vi "set_Xscale_range.vi"(8 "error in (no error)":errorcluster, 11 "Detector in":refnum<class "Detector.lvclass">) -> (0 "error out":errorcluster, 3 "Detector out":refnum<class "Detector.lvclass">)   [LabVIEW 2015, in "Detector.lvclass"]
uses:
  Detector.lvclass
  Detector.lvclass/Detector.ctl
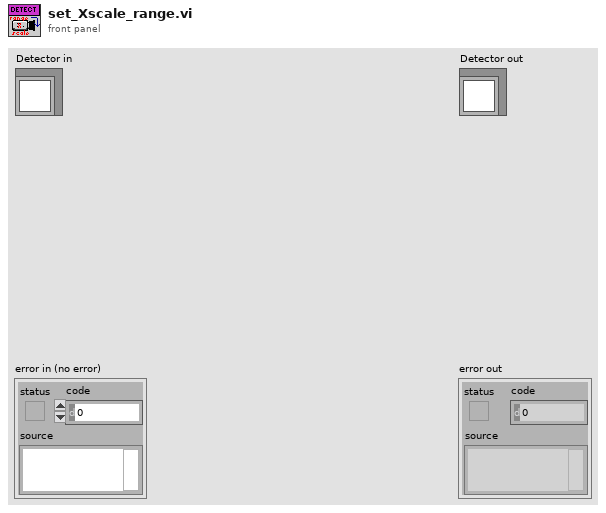
[diagram p1: front panel]
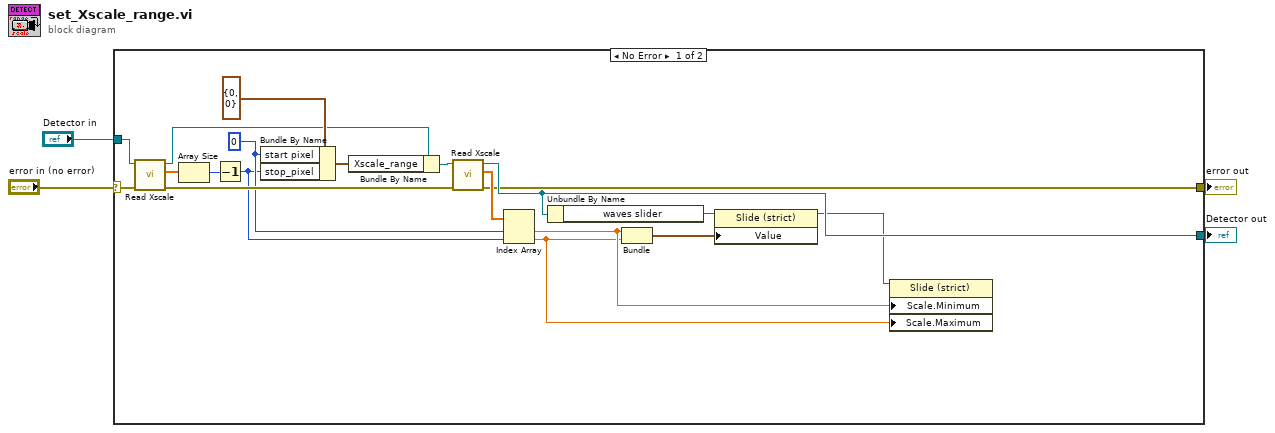
[diagram p0: block diagram]
diagram:
  n1 = case shown="No Error" "error in (no error)" {
    selector: "error in (no error)" -> [w22 w24]
    tunnel: [w8 w24] -> w3
    tunnel: [w9 w25] -> w1
    tunnel: "Detector in" -> [w23 w25]
    frame No Error {
      w12 = 0 ("start pixel")
      n2 = call "Read Xscale.vi"("error in (no error)"=w22, "Detector en entrée"=w23) -> ("error out"=w15:errorcluster, "Xscale"=w21:dbl[], "Detector en sortie"=w18:refnum<class "Detector.lvclass">)  [unwired: 7 in]
      n3 = Array Size(array=w21) -> (size(s)=w19:i32)
      n4 = Decrement(x=w19) -> (x-1=w11:i32)
      n5 = Bundle By Name(cluster=cluster{"start pixel":i32, "stop_pixel":i32} {"start pixel"=0, "stop_pixel"=0} ("Xscale_range"), "start pixel"=w12, "stop_pixel"=w11) -> (w16:cluster{"start pixel":i32, "stop_pixel":i32})
      n6 = Bundle By Name(cluster=w18, "Xscale_range"=w16) -> (w14:refnum<class "Detector.lvclass">)
      n7 = call "Read Xscale.vi"("error in (no error)"=w15, "Detector en entrée"=w14) -> ("error out"=w8:errorcluster, "Xscale"=w13:dbl[], "Detector en sortie"=w9:refnum<class "Detector.lvclass">)  [unwired: 7 in]
      n8 = Index Array(array=w13, index #1=w12, index #2=w11) -> (element #1=w6:dbl, element #2=w5:dbl)
      n9 = Unbundle By Name(w9) -> ("waves slider"=w17:refnum<vi>)
      n10 = Bundle("Numérique"=w6, "Numérique"=w5) -> (w10:cluster{"Numérique":dbl, "Numérique":dbl})  [unwired: 1 in]
      n11 = property class="Slide (strict)"(reference=w17, "Value"=w10) -> (reference out=w7:refnum<vi>)  [unwired: 1 in, 1 out]
      n12 = property class="Slide (strict)"(reference=w7, "Scale.Minimum"=w6, "Scale.Maximum"=w5) -> ()  [unwired: 1 in, 2 out]
    }
    frame Error {
    }
  }
  "error out" <- w3
  "Detector out" <- w1
